vi "lsl resolve byprop.vi"(5 "timeout":dbl, 6 "minimum":i32, 7 "value":string, 8 "error in (no error)":errorcluster, 9 "prop":string, 10 "buffer_elements":u32, 11 "buffer":cluster{}) -> (0 "error out":errorcluster, 2 "function return":i32, 3 "buffer out":cluster{})   [LabVIEW 2018, in "liblsl-LabVIEW.lvlib"]
doc: "extern LIBLSL_C_API int32_t lsl_resolve_byprop(lsl_streaminfo *buffer, uint32_t buffer_elements, const char *prop, const char *value, int32_t minimum, double timeout);"
uses:
  <userlib>/liblsl-LabVIEW/liblsl-LabVIEW.lvlib
  <userlib>/liblsl-LabVIEW/liblsl64.dll
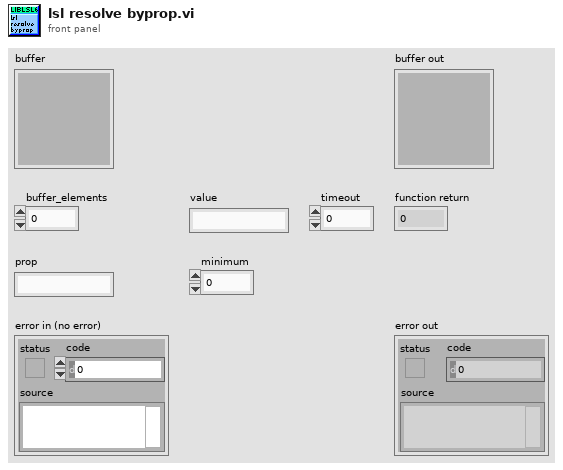
[diagram p1: front panel]
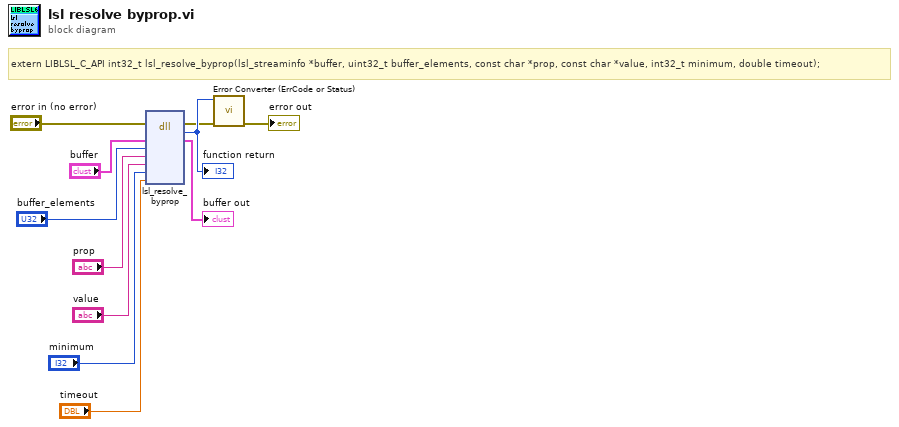
[diagram p0: block diagram]
diagram:
  # "extern LIBLSL_C_API int32_t lsl_resolve_byprop(lsl_streaminfo *buffer, uint32_t buffer_elements, const char *prop, const char *value, int32_t minimum, double timeout);"
  n1 = dll-call lib="C:/Program Files/National Instruments/LabVIEW 2018/user.lib/liblsl-LabVIEW/liblsl64.*" fn="lsl_resolve_byprop"(error in="error in (no error)", "buffer"="buffer", "buffer_elements"="buffer_elements", "prop"="prop", "value"="value", "minimum"="minimum", "timeout"="timeout") -> (error out=w2:errorcluster, w11:i32, "buffer"=→"buffer out":cluster{})  [unwired: 7 in, 1 out]
  "function return" <- w11
  n2 = call <userlib>:"Error Converter (ErrCode or Status).vi"("error in (no error)"=w2, "error code"=w11) -> ("error out"=→"error out":errorcluster)  [unwired: 9 in]
